vi "Read Arm.vi"(8 "error in (no error)":errorcluster, 11 "Fault-Injection Bus in":refnum<class "Fault-Injection Bus.lvclass">) -> (0 "error out":errorcluster, 2 "Arm":refnum<data-value>, 3 "Fault-Injection Bus out":refnum<class "Fault-Injection Bus.lvclass">)   [LabVIEW 2021, in "Fault-Injection Bus.lvclass"]
uses:
  Fault-Injection Bus.lvclass
  Fault-Injection Bus.lvclass/Fault-Injection Bus.ctl
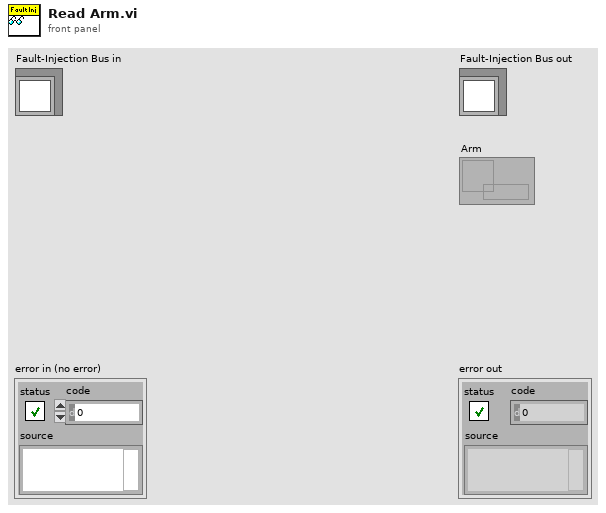
[diagram p1: front panel]
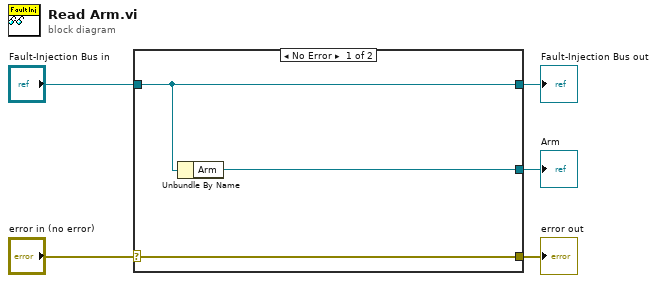
[diagram p0: block diagram]
diagram:
  n1 = case shown="No Error" "error in (no error)" {
    selector: "error in (no error)" -> [w8 w9]
    tunnel: [w8 w9] -> w4
    tunnel: [w7 w10] -> w2
    tunnel: "Fault-Injection Bus in" -> [w7 w10]
    tunnel: [w6 _] -> w1
    frame No Error {
      n2 = Unbundle By Name(w7) -> ("Arm"=w6:refnum<data-value>)
    }
    frame Error {
    }
  }
  "error out" <- w4
  "Fault-Injection Bus out" <- w2
  "Arm" <- w1
